vi "Init.vi"(8 "error in":errorcluster, 11 "Column Header in":refnum<class "Column Header.lvclass">) -> (0 "error out":errorcluster, 3 "Column Header out":refnum<class "Column Header.lvclass">)   [LabVIEW 2023, in "SourceGrid.lvlib" / "Column Header.lvclass"]
uses:
  Column Header.lvclass
  D:/git/Sourcegrid-LabVIEW/dll/SourceGrid.dll
  dll/SourceGrid.dll
  Cell/Cell.lvclass
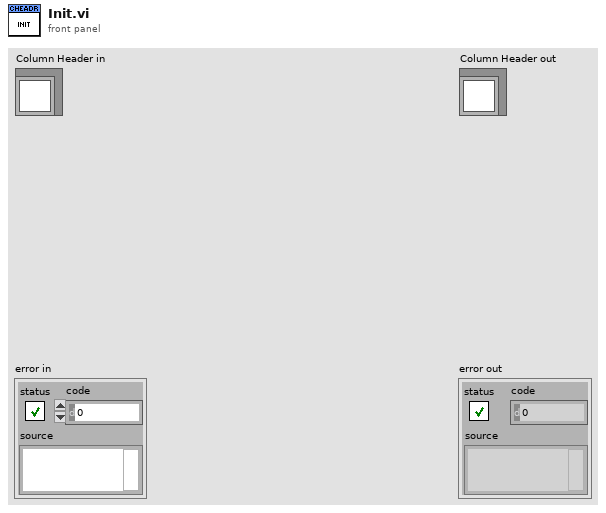
[diagram p1: front panel]
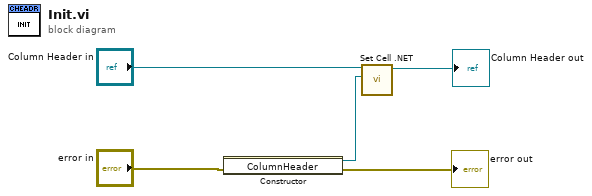
[diagram p0: block diagram]
diagram:
  n1 = constructor class="ColumnHeader"(error in="error in") -> (reference out=w1:refnum<k24>, error out=→"error out":errorcluster)  [unwired: 2 in, 1 out]
  n2 = call "Set Cell .NET.vi"("Cell .NET"=w1, "Cell in"="Column Header in") -> ("Cell out"=→"Column Header out":refnum<class "Column Header.lvclass">)  [unwired: 9 in]
